vi "Load Sub Panel.vi"(8 "error in (no error)":errorcluster, 10 "sub panel":refnum<vi>, 11 "Log in":refnum<class "Log.lvclass">) -> (0 "error out":errorcluster, 3 "Log out":refnum<class "Log.lvclass">)   [LabVIEW 2020, in "Log.lvlib" / "Log.lvclass"]
uses:
  Log.lvclass
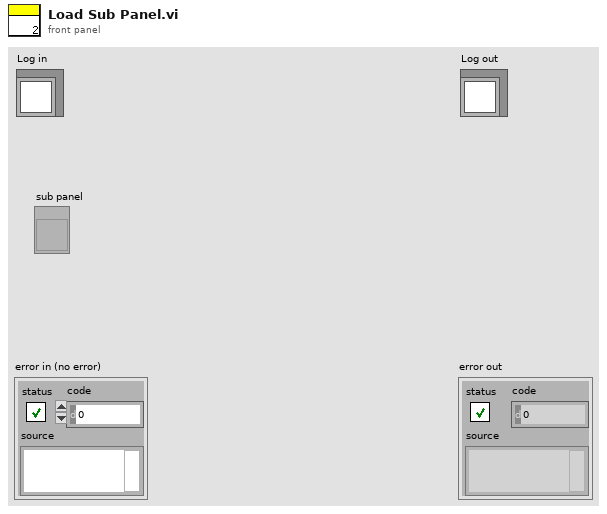
[diagram p1: front panel]
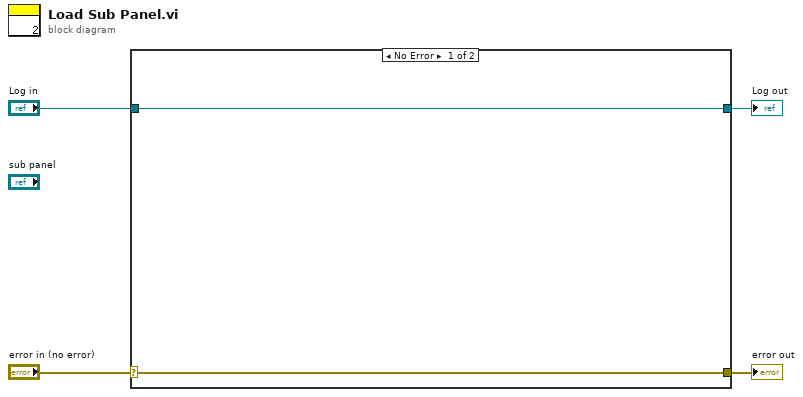
[diagram p0: block diagram]
diagram:
  n1 = case shown="No Error" "error in (no error)" {
    selector: "error in (no error)" -> [w5 w8]
    tunnel: [w5 w8] -> w3
    tunnel: [w6 w7] -> w1
    tunnel: "Log in" -> [w6 w7]
    frame No Error {
    }
    frame Error {
    }
  }
  "error out" <- w3
  "Log out" <- w1
